vi "Flywheel Moment of Inertia.vi"(8 "Gear Ratio (out/in)":dbl=0.2, 11 "Flywheel Coefficients":T2={"Mass"=0.45359237, "Radius"=0.1, "Coefficient (https://en.wikipedia.org/wiki/List_of_moments_of_inertia)"=0.5, "Name"=""}) -> (0 "Physical Values":T1 {"Moment of Inertia (kg m^2)" format="%#_3p"})   [LabVIEW 2019]
uses:
  Motor Physical Values.ctl
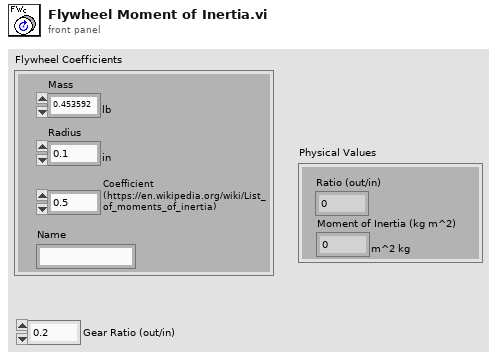
[diagram p1: front panel]
types:
  T1 = typedef "Motor Physical Values.ctl" = cluster{"Ratio (out/in)":dbl, "Moment of Inertia (kg m^2)":dbl[unit]}
  T2 = cluster{"Mass":dbl[unit], "Radius":dbl[unit], "Coefficient (https://en.wikipedia.org/wiki/List_of_moments_of_inertia)":dbl, "Name":string}
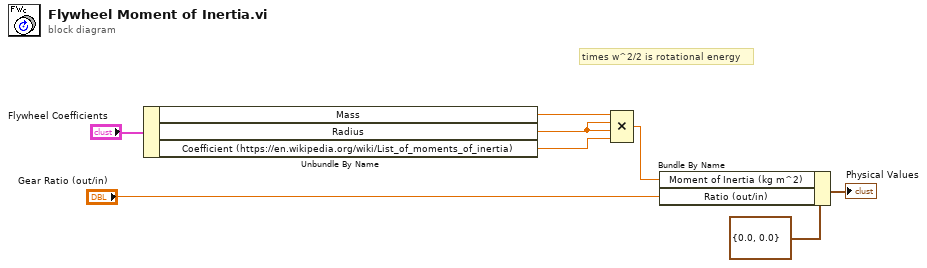
[diagram p0: block diagram]
diagram:
  # "times w^2/2 is rotational energy"
  n1 = Unbundle By Name("Flywheel Coefficients") -> ("Mass"=w7:dbl[unit], "Radius"=w6:dbl[unit], "Coefficient (https://en.wikipedia.org/wiki/List_of_moments_of_inertia)"=w5:dbl)
  n2 = Compound Arithmetic op=MULTIPLY(w7, w6, w6, w5) -> (w2:dbl[unit])
  n3 = Bundle By Name(cluster=T1 {"Ratio (out/in)"=0.0, "Moment of Inertia (kg m^2)"=0.0} ("Physical Values"), "Moment of Inertia (kg m^2)"=w2, "Ratio (out/in)"="Gear Ratio (out/in)") -> (→"Physical Values":T1)
